vi "Set Panel Controller_Q.vi"(8 "error in (no error)":errorcluster, 10 "Panel Controller_Q":refnum<class "Message Enqueuer.lvclass">, 11 "Panel Control_Ref in":refnum<class "Panel Controller.lvclass">) -> (0 "error out":errorcluster, 3 "Panel Control_Ref out":refnum<class "Panel Controller.lvclass">)   [LabVIEW 2015, in "Panel Controller.lvclass"]
uses:
  Panel Controller.lvclass
  <vilib>/ActorFramework/Message Enqueuer/Message Enqueuer.lvclass
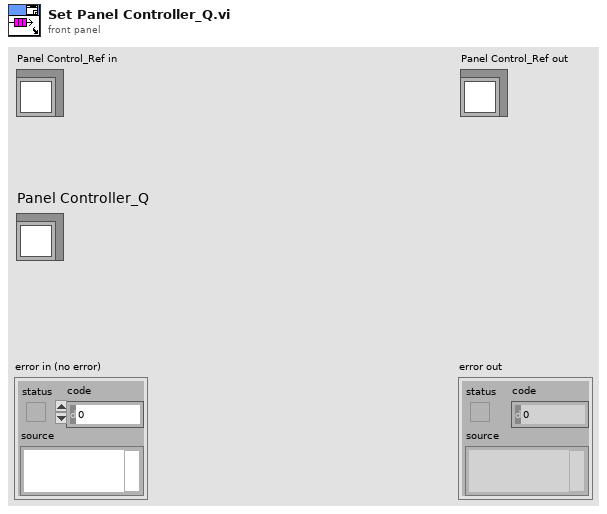
[diagram p1: front panel]
types:
  T1 = typedef "Panel Controller.lvclass/ObjectAttributes.ctl" = cluster{"Sub Panel Ref":refnum<vi>, "Panel_Q":refnum<queue>, "VI Running Refnum":refnum<vi>, "Brower Controller_Q":refnum<class "Message Enqueuer.lvclass">, "GUI Control Builder Director.lvclass":refnum<class "GUI Control Builder Director.lvclass">, "Panel GUI Manager.lvclass":refnum<class "Panel GUI Manager.lvclass">}
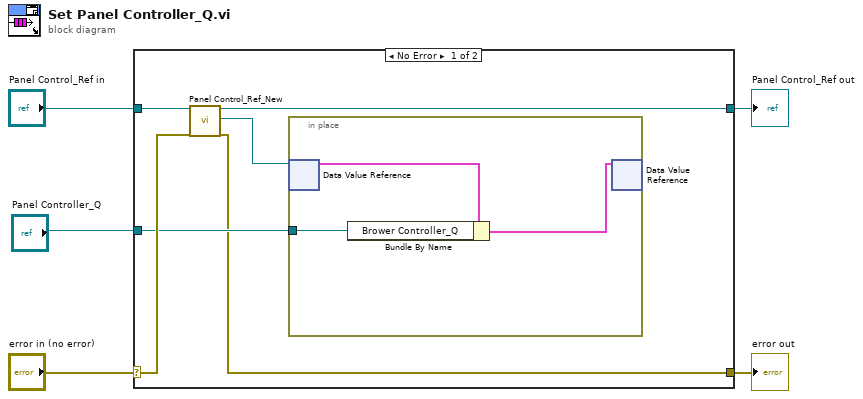
[diagram p0: block diagram]
diagram:
  n1 = case shown="No Error" "error in (no error)" {
    selector: "error in (no error)" -> [w10 w16]
    tunnel: [w6 w16] -> w4
    tunnel: [w7 w15] -> w2
    tunnel: "Panel Control_Ref in" -> [w11 w15]
    tunnel: "Panel Controller_Q" -> [w8 _]
    frame No Error {
      n2 = call "Panel Control_Ref_New.vi"("reference in"=w11, "error in (no error)"=w10) -> ("reference out"=w7:refnum<class "Panel Controller.lvclass">, "DVRRefOut"=w9:refnum<data-value>, "error out"=w6:errorcluster)  [unwired: 14 in, 1 out]
      n3 = in-place {
        in-place-border: w8 -> [w13]
        n4 = in-place-dvr #1(w9) -> (w14:T1)  [unwired: 1 out]
        n5 = Bundle By Name(cluster=w14, "Brower Controller_Q"=w13) -> (w12:T1)
        n6 = in-place-dvr #1(w12) -> ()  [unwired: 2 out]
      }
    }
    frame Error {
    }
  }
  "error out" <- w4
  "Panel Control_Ref out" <- w2
